vi "Get SubVI References (by Pattern).vi"(8 "error in (no error)":errorcluster, 10 "SubVI Name Pattern":string, 11 "VI ref in":refnum<vi>) -> (0 "error out":errorcluster, 2 "SubVI refs":refnum<vi>[](array[refnum]), 3 "VI ref out":refnum<vi>)   [LabVIEW 2019, in "gRPC Template Creation Utility.lvlib"]
uses:
  gRPC Template Creation Utility.lvlib
  <vilib>/Utility/traverseref.llb/TRef TravTarget.ctl
  <vilib>/Utility/traverseref.llb/VI Scripting - Traverse.lvlib
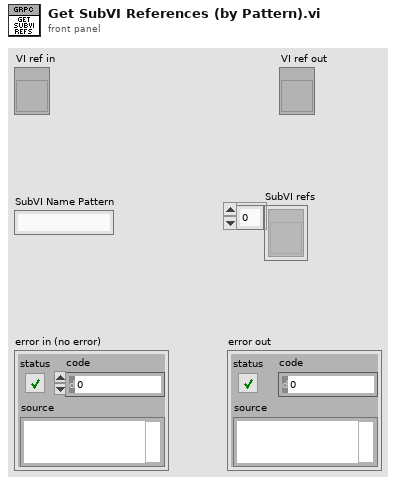
[diagram p1: front panel]
types:
  T1 = typedef "TRef TravTarget.ctl" = enum16{"FP", "BD", "Other"}
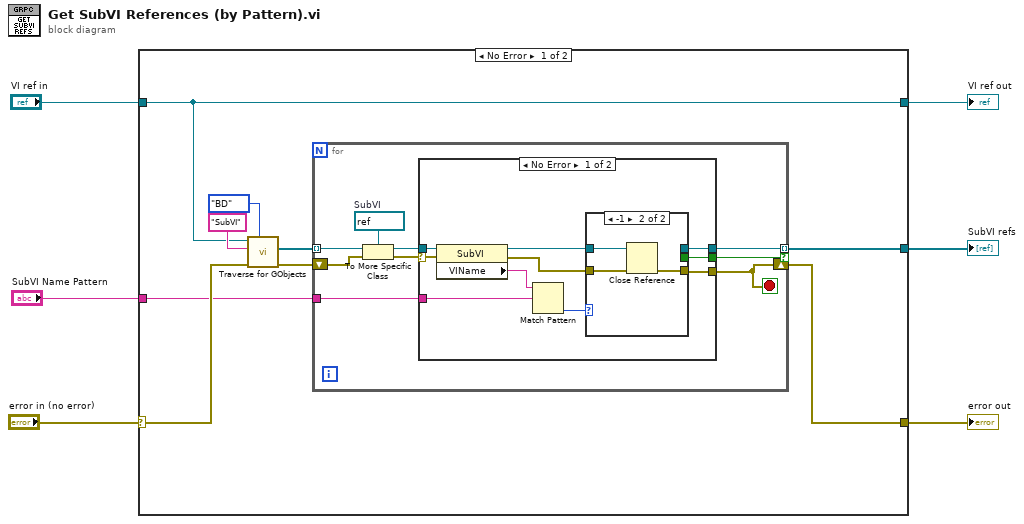
[diagram p0: block diagram]
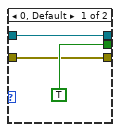
[diagram p2: hidden frame]
diagram:
  n1 = case shown="No Error" "error in (no error)" {
    selector: "error in (no error)" -> [w10 w44]
    tunnel: [w15 _] -> w6
    tunnel: "VI ref in" -> [w8 w43]
    tunnel: [w9 w44] -> w1
    tunnel: [w8 w43] -> w3
    tunnel: "SubVI Name Pattern" -> [w7 _]
    frame No Error {
      n2 = call <vilib>:"Traverse for GObjects.vi"("Traverse Target"=TRef_TravTarget."BD", "error in (no error)"=w10, "Class Name"="SubVI", "VI Refnum"=w8) -> ("error out"=w13:errorcluster, "References"=w12:refnum<vi>[])  [unwired: 4 in, 2 out]
      n3 = for {
        tunnel: w12 -> [w24] mode=indexing
        tunnel: [w20] -> w15 mode=indexing if=w19
        shift-right: [w17] -> w9
        shift-left: w13 -> [w22]
        tunnel: w7 -> [w18]
        stop <- w17 stop-if-true
        w23 = refnum<vi> refnum  # SubVI
        n4 = To More Specific Class(target class=w23, reference=w24, error in=w22) -> (specific class reference=w21:refnum<vi>, error out=w16:errorcluster)
        n5 = case shown="No Error" w16 {
          selector: w16 -> [w25 w42]
          tunnel: w21 -> [w34 w41]
          tunnel: [w29 w41] -> w20
          tunnel: [w28 _] -> w19
          tunnel: w18 -> [w27 _]
          tunnel: [w26 w42] -> w17
          frame No Error {
            n6 = property class="SubVI"(reference=w34, error in=w25) -> (reference out=w31:refnum<vi>, error out=w30:errorcluster, "VIName"=w33:string)
            n7 = Match Pattern(string=w33, regular expression=w27) -> (offset past match=w32:i32)  [unwired: 1 in, 3 out]
            n8 = case shown="-1" w32 {
              tunnel: w31 -> [w37 w40]
              tunnel: w30 -> [w35 w39]
              tunnel: [w37 _] -> w29
              tunnel: [TRUE _] -> w28
              tunnel: [w35 w38] -> w26
              frame 0, Default {
              }
              frame -1 {
                n9 = Close Reference(reference=w40, error in (no error)=w39) -> (error out=w38:errorcluster)
              }
            }
          }
          frame Error {
          }
        }
      }
    }
    frame Error {
    }
  }
  "SubVI refs" <- w6
  "VI ref out" <- w3
  "error out" <- w1
